vi "New0002.vi"   [LabVIEW 2013]
uses:
  <vilib>/Heliosphere Research LLC/Advanced Plotting Toolkit/Advanced Plotting Toolkit.lvlib
types:
  T1 = typedef "Advanced Plotting Toolkit.lvlib/PlotID.ctl" = i32
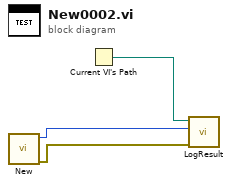
[diagram p0: block diagram]
diagram:
  n1 = call <vilib>:"New.vi"() -> ("error out"=w1:errorcluster, "Plot ID"=w2:T1)  [unwired: 10 in]
  n2 = Current VI's Path() -> (path=w3:path)
  n3 = call "LogResult.vi"("Test Result"=w1, "Test Artifact"=w2, "VI Path"=w3) -> ()  [unwired: 9 in]
